vi "Acq Get Properties.vi"(0 "session in":refnum<class "Digitizer Control.lvclass">, 5 "error in (no error)":errorcluster) -> (13 "maximum pre-trigger period (s)":dbl, 14 "session out":refnum<class "Digitizer Control.lvclass">, 19 "error out":errorcluster)   [LabVIEW 2021, in "Digitizer Control.lvclass"]
doc: "Returns acquisition session properties.\n\nInputs:\n\n<B>session in</B>: The device session.\n\nOutputs:\n\n<B>session out</B>: The device session passed on the <B>session in</B> input.\n\n<B>maximum pre-trigger period (s)</B>: The pre-trigger period is the period acquired before recognizing the start trigger. This output returns the maximum pre-trigger period, in seconds, supported by the device."
uses:
  Digitizer Control.lvclass
  Digitizer Control.lvclass/Digitizer Control.ctl
  <vilib>/Utility/error.llb/Error Cluster From Error Code.vi
  <vilib>/rvi/errors/niLvFpgaAdjustHostInterfaceError.vi
  <vilib>/rvi/interface/nirviReadWriteControl/nirviReadWriteControl.xnode
  NiFpgaLv.dll
  <vilib>/rvi/interface/Simulation/niFpgaSimulationCallBeginRW.vi
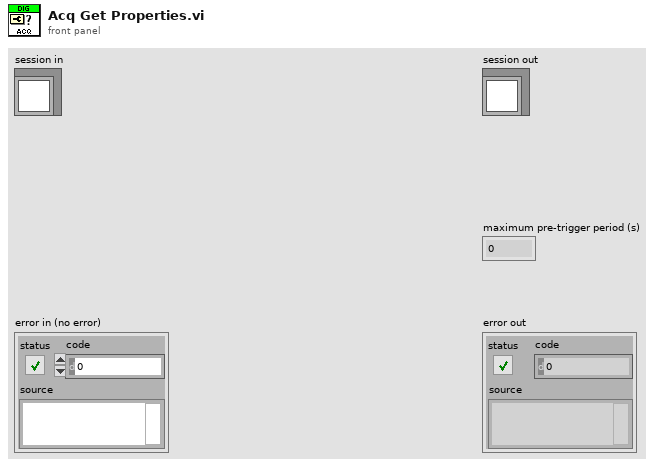
[diagram p1: front panel]
types:
  T1 = typedef "Digitizer Control.lvclass/Acq Session Data.ctl" = cluster{"ADC sampling rate":dbl, "SCTL rate":dbl, "DMA element size (bits)":i32, "sample size (bits)":i32[], "DMA/memory interface width (DMA elements)":i32, "transfer size (bits)":i32[], "stream instance":i32[], "trigger instance":u32, "group delay (s)":dbl, "data delay (s)":dbl, "target delay (s)":dbl, "trigger tracking enabled":bool, "channel configured":bool, "enabled channels":bool[], "transfer configured":bool, "dsp bypass":bool, "fractional decimator input rate":dbl, "fractional decimator output rate":dbl, "sample scale factor":dbl[], "memory size":u64[], "FIFO size":u64}
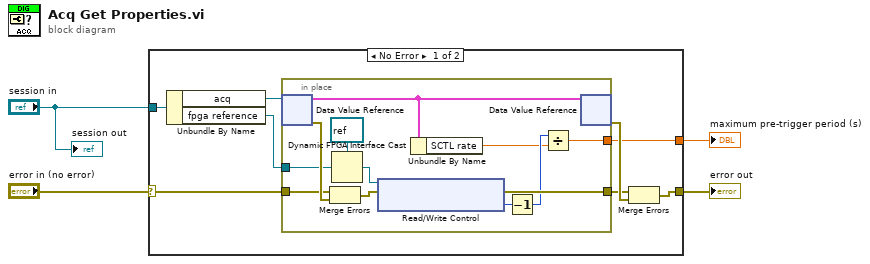
[diagram p0: block diagram]
diagram:
  n1 = case shown="No Error" "error in (no error)" {
    selector: "error in (no error)" -> [w11 w25]
    tunnel: [w9 w25] -> w3
    tunnel: "session in" -> [w8 _]
    tunnel: [w5 _] -> w1
    frame No Error {
      n2 = Unbundle By Name(w8) -> ("acq"=w7:refnum<data-value>, "fpga reference"=w6:refnum<k20>)
      n3 = in-place {
        in-place-border: [w18] -> w10
        in-place-border: w11 -> [w22]
        in-place-border: w6 -> [w21]
        in-place-border: [w13] -> w5
        n4 = in-place-dvr #1(w7) -> (w17:T1, w24:errorcluster)
        n5 = Merge Errors(w22, w24) -> (w20:errorcluster)
        n6 = Dynamic FPGA Interface Cast(Session In=refnum<k20> refnum ("FPGA Interface"), Type=w21) -> (Session Out=w19:refnum<k20>)
        n7 = xnode "Read/Write Control"("FPGA VI Reference In"=w19, "error in"=w20) -> ("error out"=w18:errorcluster, "acq.maximum delay"=w16:u16)  [unwired: 1 out]
        n8 = Unbundle By Name(w17) -> ("SCTL rate"=w14:dbl)
        n9 = Decrement(x=w16) -> (x-1=w15:u16)
        n10 = Divide(x=w15, y=w14) -> (x/y=w13:dbl)
        n11 = in-place-dvr #1(w17) -> (w12:errorcluster)  [unwired: 1 out]
      }
      n12 = Merge Errors(w10, w12) -> (w9:errorcluster)
    }
    frame Error {
    }
  }
  "error out" <- w3
  "maximum pre-trigger period (s)" <- w1
  "session out" <- "session in"
